vi "proc_terminate.vi"(7 "timeout [ms]":i32, 8 "error in":errorcluster, 11 "process instance handle in":u32[](array[numeric])) -> (0 "error out":errorcluster, 3 "process instance handle out":u32[](array[numeric]))   [LabVIEW 2011]
doc: "Tries to kill process instance (TerminateProcess). If it is successful, waits for actual termination and closes process instance handle.\nThis VI is recommended to use only if there is no other way how to force process exit. For example GNU Octave can be closed by \"exit\" command."
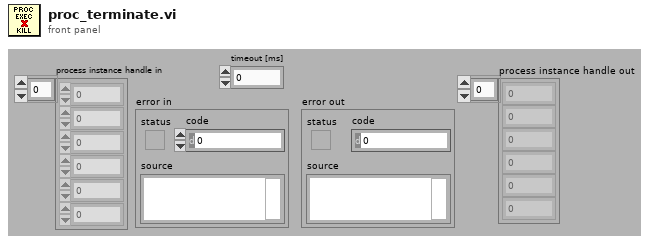
[diagram p1: front panel]
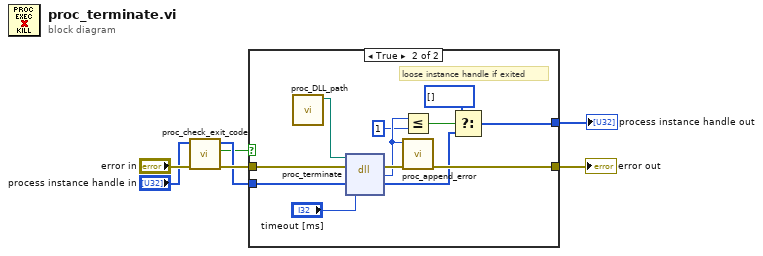
[diagram p0: block diagram]
diagram:
  n1 = call "proc_check_exit_code.vi"("error in"="error in", "instance handle in"="process instance handle in") -> ("error out"=w5:errorcluster, "running"=w1:bool, "instance handle out"=w3:u32[])  [unwired: 5 in, 2 out]
  n2 = case shown="True" w1 {
    tunnel: [w8 w21] -> w7
    tunnel: w5 -> [w8 w20]
    tunnel: w3 -> [w9 w19]
    tunnel: [w9 w12] -> w2
    frame False {
    }
    frame True {
      # "loose instance handle if exited"
      n3 = call "proc_DLL_path.vi"() -> ("path out"=w18:path)  [unwired: 10 in, 1 out]
      n4 = dll-call lib="lv_proc.dll" fn="proc_terminate"(path in=w18, error in=w20, "proc"=w19, "timeout [ms]"="timeout [ms]") -> (error out=w17:errorcluster, "error"=w15:i32, "proc"=w11:u32[])  [unwired: 2 in, 1 out]
      n5 = Less Or Equal?(x=w15, y=1) -> (x <= y?=w13:bool)
      n6 = call "proc_append_error.vi"("error in"=w17, "code in"=w15) -> ("error out"=w21:errorcluster)  [unwired: 8 in, 1 out]
      n7 = Select(t=u32[] [], s=w13, f=w11) -> (s? t:f=w12:u32[])
    }
  }
  "error out" <- w7
  "process instance handle out" <- w2
